vi "get 750 mag stable.vi"(10 "类型":enum16{"temp", "field", "position"}(ring), 11 "输出簇":T1={"initialize"=enum."SR830", "6221"={"6221 Resource"="GPIB0::24::INSTR", "Delta status"=FALSE, "电流|RMS(A)"=0.0}, "SR830+6221"={"source"=0, "Current(A)"=0.0, "阻抗(Ohm)"=0.0, "SR830 1"=FALSE, "SR830 2"=FALSE, "SR830 3"=FALSE, "SR830 4"=FALSE, "VISA 1"="", "VISA 2"="", "VISA 3"="", "VISA 4"="", "Reserve 1"=0, "Reserve 2"=-1, "Reserve 3"=-1, "Reserve 4"=-1, "Sensitivity 1"=-1, "Sensitivity 2"=0, "Sensitivity 3"=-1, "Sensitivity 4"=-1, "量程入 1"=0, "量程入 2"=0, "量程入 3"=0, "量程入 4"=0}, "2400"={"2400"=FALSE, "VISA"="", "Output Level (0)"=1e-05, "Compliance  Level (0.1)"=10.0}, "ch"={"ch"=[], "current"=[], "change?"=[], "holding current\nwhen change ch?"=FALSE}, "Instrument"={"325 Resource "="GPIB0::13::INSTR", "Input (0:A) 325"=0, "Heater Output (1:1) 325"=1, "340 Resource"="GPIB0::14::INSTR", "Input (0:A) 340"=0, "Loop (0: 1)"=0, "Input (0:B) 340"=1, "Loop (1: 1)"=0, "340 Status"=refnum, "Instrument Type"=enum."PPMS-Rotate", "quantum design"=refnum, "semaphore 325"=refnum, "TCP master instance"=refnum, "M24C Resource"="GPIB0::24::INSTR", "4G supply"="GPIB0::24::INSTR", "Temp Status 24C"=refnum, "Temp"=refnum, "9T信号"=refnum, "limit"={"Field limit"=0.0, "Field rate limit"=0.0, "Temp limit"=0.0, "Temp low limit"=0.0, "Temp rate limit "=0.0}, "4g supply status"=refnum, "vi路径"="", "in-plane"="", "out-plane"="", "in-plane signal"=FALSE, "out-plane signal"=FALSE, "in plane 信号"=refnum, "pzt volt"=refnum, "Aborting"=refnum, "数据文件"=refnum, "warning"=refnum, "750 visa"="", "750 rotate"="", "335 Status 2"=refnum, "335 Resource "="GPIB0::24::INSTR", "Input (0:A) 335"=0, "Input (0:B) 335"=1, "Heater Output (1:1) 335"=1, "semaphore 340"=refnum, "semaphore 335"=refnum, "325 Status"=refnum, "semaphore 750"=refnum, "750 field status"=refnum, "camg 振荡状态"=refnum, "列表框"=refnum, "编辑列表框？"=refnum, "camg Rate"=refnum, "行数"=refnum, "TM620"="TCPIP0::192.168.1.5::4266::SOCKET"}, "2614B"={"2614B chA"=FALSE, "2614B chB"=FALSE, "VISA"=""}, "33522b"={"33522b resource name"="", "零电压"=0.0, "最大电压"=148.0, "间隔"=4.0, "最小电压"=-48.0, "PZT Scan?"=FALSE}, "gating type"=enum."2614(daul)", "层数"=0, "行数"=0, "是否处理"=[]} {"Instrument"."Loop (1: 1)" items=["1"=1, "2"=2]; "Instrument"."Loop (0: 1)" items=["1"=1, "2"=2]; "Instrument"."Input (0:B) 340" items=["A", "B", "C", "D"]; "Instrument"."Heater Output (1:1) 335" items=["1"=1, "2"=2]; "Instrument"."Input (0:B) 335" items=["A", "B"]; "Instrument"."Input (0:A) 335" items=["A", "B"]; "Instrument"."Heater Output (1:1) 325" items=["1"=1, "2"=2]; "Instrument"."Input (0:A) 325" items=["A", "B"]; "Instrument"."Input (0:A) 340" items=["1"=1, "2"=2]; "SR830+6221"."Sensitivity 4" items=["Auto Gain"=-1, "2 nV/fA"=0, "5 nV/fA"=1, "10 nV/fA"=2, "20 nV/fA"=3, "50 nV/fA"=4, "100 nV/fA"=5, "200 nV/fA"=6, "500 nV/fA"=7, "1 uV/pA"=8, "2 uV/pA"=9, "5 uV/pA"=10, "10 uV/pA"=11, "20 uV/pA"=12, "50 uV/pA"=13, "100 uV/pA"=14, "200 uV/pA"=15, "500 uV/pA"=16, "1 mV/nA"=17, "2 mV/nA"=18, "5 mV/nA"=19, "10 mV/nA"=20, "20 mV/nA"=21, "50 mV/nA"=22, "100 mV/nA"=23, "200 mV/nA"=24, "500 mV/mA"=25, "1 V/uA"=26]; "SR830+6221"."Sensitivity 3" items=["Auto Gain"=-1, "2 nV/fA"=0, "5 nV/fA"=1, "10 nV/fA"=2, "20 nV/fA"=3, "50 nV/fA"=4, "100 nV/fA"=5, "200 nV/fA"=6, "500 nV/fA"=7, "1 uV/pA"=8, "2 uV/pA"=9, "5 uV/pA"=10, "10 uV/pA"=11, "20 uV/pA"=12, "50 uV/pA"=13, "100 uV/pA"=14, "200 uV/pA"=15, "500 uV/pA"=16, "1 mV/nA"=17, "2 mV/nA"=18, "5 mV/nA"=19, "10 mV/nA"=20, "20 mV/nA"=21, "50 mV/nA"=22, "100 mV/nA"=23, "200 mV/nA"=24, "500 mV/mA"=25, "1 V/uA"=26]; "SR830+6221"."Sensitivity 1" items=["Auto Gain"=-1, "2 nV/fA"=0, "5 nV/fA"=1, "10 nV/fA"=2, "20 nV/fA"=3, "50 nV/fA"=4, "100 nV/fA"=5, "200 nV/fA"=6, "500 nV/fA"=7, "1 uV/pA"=8, "2 uV/pA"=9, "5 uV/pA"=10, "10 uV/pA"=11, "20 uV/pA"=12, "50 uV/pA"=13, "100 uV/pA"=14, "200 uV/pA"=15, "500 uV/pA"=16, "1 mV/nA"=17, "2 mV/nA"=18, "5 mV/nA"=19, "10 mV/nA"=20, "20 mV/nA"=21, "50 mV/nA"=22, "100 mV/nA"=23, "200 mV/nA"=24, "500 mV/mA"=25, "1 V/uA"=26]; "SR830+6221"."Sensitivity 2" items=["Auto Gain"=-1, "2 nV/fA"=0, "5 nV/fA"=1, "10 nV/fA"=2, "20 nV/fA"=3, "50 nV/fA"=4, "100 nV/fA"=5, "200 nV/fA"=6, "500 nV/fA"=7, "1 uV/pA"=8, "2 uV/pA"=9, "5 uV/pA"=10, "10 uV/pA"=11, "20 uV/pA"=12, "50 uV/pA"=13, "100 uV/pA"=14, "200 uV/pA"=15, "500 uV/pA"=16, "1 mV/nA"=17, "2 mV/nA"=18, "5 mV/nA"=19, "10 mV/nA"=20, "20 mV/nA"=21, "50 mV/nA"=22, "100 mV/nA"=23, "200 mV/nA"=24, "500 mV/mA"=25, "1 V/uA"=26]; "SR830+6221"."Reserve 4" items=["Auto Gain"=-1, "2 nV/fA"=0, "5 nV/fA"=1, "10 nV/fA"=2, "20 nV/fA"=3, "50 nV/fA"=4, "100 nV/fA"=5, "200 nV/fA"=6, "500 nV/fA"=7, "1 uV/pA"=8, "2 uV/pA"=9, "5 uV/pA"=10, "10 uV/pA"=11, "20 uV/pA"=12, "50 uV/pA"=13, "100 uV/pA"=14, "200 uV/pA"=15, "500 uV/pA"=16, "1 mV/nA"=17, "2 mV/nA"=18, "5 mV/nA"=19, "10 mV/nA"=20, "20 mV/nA"=21, "50 mV/nA"=22, "100 mV/nA"=23, "200 mV/nA"=24, "500 mV/mA"=25, "1 V/uA"=26]; "SR830+6221"."Reserve 3" items=["Auto Reserve"=-1, "High Reserve"=0, "Normal"=1, "Low Noise"=2]; "SR830+6221"."Reserve 2" items=["Auto Reserve"=-1, "High Reserve"=0, "Normal"=1, "Low Noise"=2]; "SR830+6221"."Reserve 1" items=["Auto Reserve"=-1, "High Reserve"=0, "Normal"=1, "Low Noise"=2]; "SR830+6221"."source" items=["SR830 1", "SR830 2", "SR830 3", "SR830 4"]}) -> (1 "Stable?":bool)   [LabVIEW 2019, in "User lib.lvlib"]
uses:
  User lib.lvlib
  ctl/config.ctl
  <vilib>/NI/Modbus Library/API/Master/Modbus Master.lvclass
  ctl/initialize.ctl
  ctl/Instrument.ctl
  ctl/335 state.ctl
  ctl/Instrument Type.ctl
  lib/QDInstrument.dll
  ctl/limit.ctl
  ctl/9T mag field stauts.ctl
  ctl/warning.ctl
  ctl/Gating type.ctl
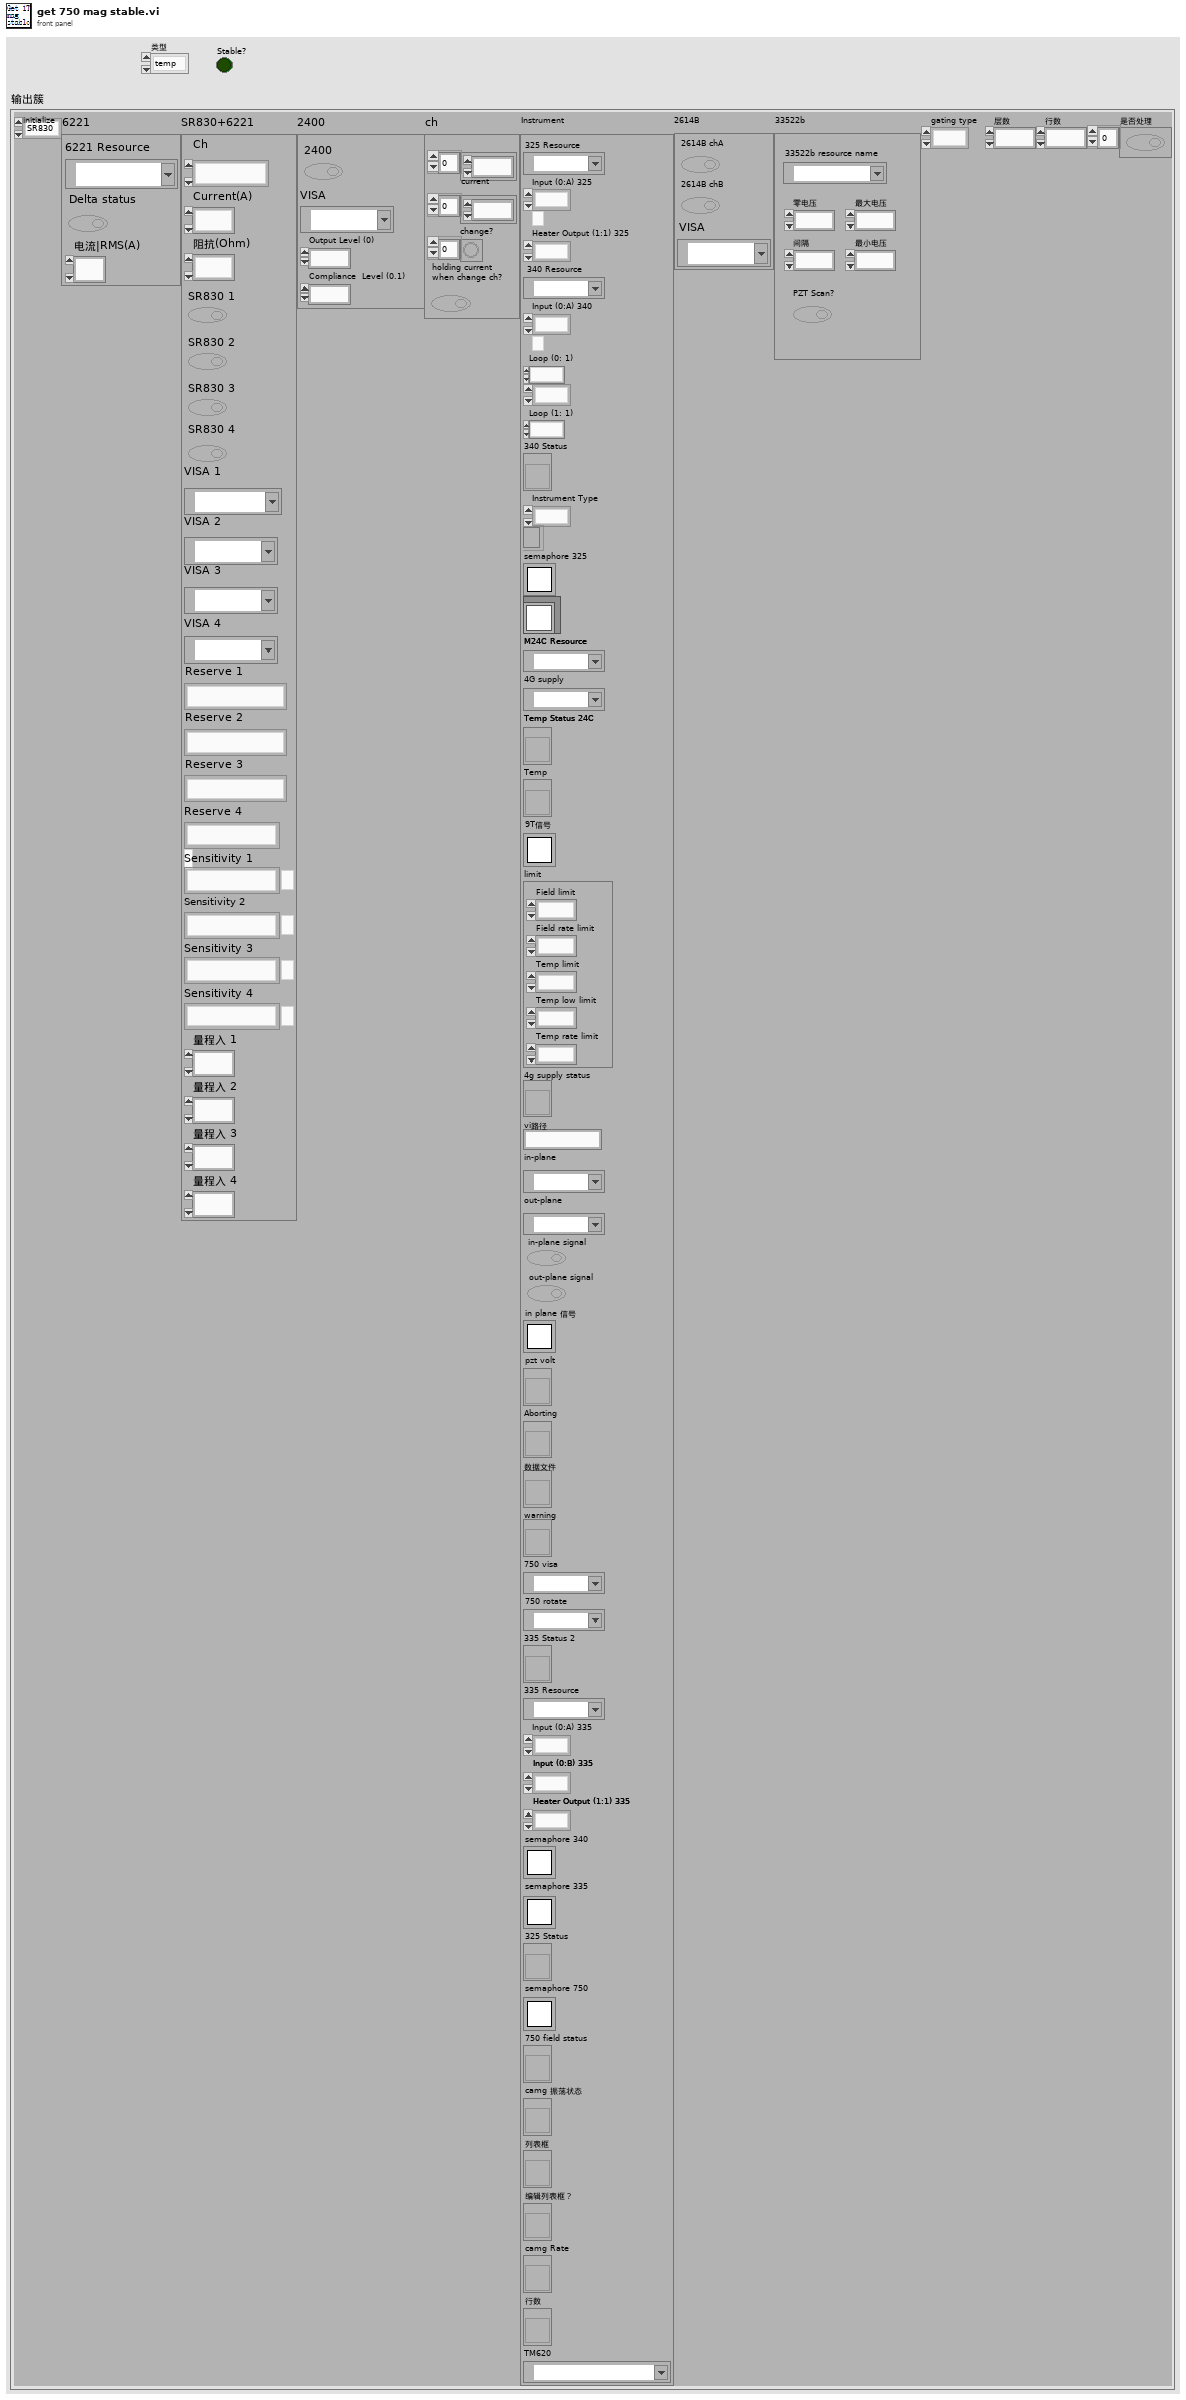
[diagram p1: front panel]
types:
  T1 = typedef "config.ctl" = cluster{"initialize":T2, "6221":cluster{"6221 Resource":refnum<visa-resource-name>, "Delta status":bool, "电流|RMS(A)":dbl}, "SR830+6221":cluster{"source":u16, "Current(A)":dbl, "阻抗(Ohm)":dbl, "SR830 1":bool, "SR830 2":bool, "SR830 3":bool, "SR830 4":bool, "VISA 1":refnum<visa-resource-name>, "VISA 2":refnum<visa-resource-name>, "VISA 3":refnum<visa-resource-name>, "VISA 4":refnum<visa-resource-name>, "Reserve 1":i16, "Reserve 2":i16, "Reserve 3":i16, "Reserve 4":i16, "Sensitivity 1":i16, "Sensitivity 2":i16, "Sensitivity 3":i16, "Sensitivity 4":i16, "量程入 1":i32, "量程入 2":i32, "量程入 3":i32, "量程入 4":i32}, "2400":cluster{"2400":bool, "VISA":refnum<visa-resource-name>, "Output Level (0)":dbl, "Compliance  Level (0.1)":dbl}, "ch":cluster{"ch":i32[], "current":dbl[], "change?":bool[], "holding current\nwhen change ch?":bool}, "Instrument":T3, "2614B":cluster{"2614B chA":bool, "2614B chB":bool, "VISA":refnum<visa-resource-name>}, "33522b":cluster{"33522b resource name":refnum<visa-resource-name>, "零电压":dbl, "最大电压":dbl, "间隔":dbl, "最小电压":dbl, "PZT Scan?":bool}, "gating type":T7, "层数":i32, "行数":i32, "是否处理":bool[]}
  T2 = typedef "initialize.ctl" = enum16{"SR830", "keithley6221-SR830", "Delta", "Delta-tunnelling", "keithley6221-2182-DC", "PZT", "4200"}
  T3 = typedef "Instrument.ctl" = cluster{"325 Resource ":refnum<visa-resource-name>, "Input (0:A) 325":u16, "Heater Output (1:1) 325":u16, "340 Resource":refnum<visa-resource-name>, "Input (0:A) 340":u16, "Loop (0: 1)":u16, "Input (0:B) 340":u16, "Loop (1: 1)":u16, "340 Status":refnum<vi>, "Instrument Type":T4, "quantum design":refnum<k24>, "semaphore 325":T5, "TCP master instance":refnum<class "Modbus Master.lvclass">, "M24C Resource":refnum<visa-resource-name>, "4G supply":refnum<visa-resource-name>, "Temp Status 24C":refnum<vi>, "Temp":refnum<vi>, "9T信号":T5, "limit":T6, "4g supply status":refnum<vi>, "vi路径":string, "in-plane":refnum<visa-resource-name>, "out-plane":refnum<visa-resource-name>, "in-plane signal":bool, "out-plane signal":bool, "in plane 信号":T5, "pzt volt":refnum<vi>, "Aborting":refnum<vi>, "数据文件":refnum<vi>, "warning":refnum<vi>, "750 visa":refnum<visa-resource-name>, "750 rotate":refnum<visa-resource-name>, "335 Status 2":refnum<vi>, "335 Resource ":refnum<visa-resource-name>, "Input (0:A) 335":u16, "Input (0:B) 335":u16, "Heater Output (1:1) 335":u16, "semaphore 340":T5, "semaphore 335":T5, "325 Status":refnum<vi>, "semaphore 750":T5, "750 field status":refnum<vi>, "camg 振荡状态":refnum<vi>, "列表框":refnum<vi>, "编辑列表框？":refnum<vi>, "camg Rate":refnum<vi>, "行数":refnum<vi>, "TM620":refnum<visa-resource-name>}
  T4 = typedef "Instrument Type.ctl" = enum16{"PPMS", "VersaLab", "DynaCool", "SVSM", "PPMS-Rotate", "Lakeshore335", "lengtou2", "9T mag old", "9T cmag", "9T cmag DAC", "9T cmag rotate", "test"}
  T5 = typedef "Semaphore RefNum" = refnum<k1>
  T6 = typedef "limit.ctl" = cluster{"Field limit":dbl, "Field rate limit":dbl, "Temp limit":dbl, "Temp low limit":dbl, "Temp rate limit ":dbl}
  T7 = typedef "Gating type.ctl" = enum32{"null", "2614(daul)", "2400", "6517B"}
  T8 = typedef "335 state.ctl" = u16
  T9 = typedef "9T mag field stauts.ctl" = enum16{"unknow", "Stable", "Sweep up", "Sweep down", "Sweep to zero", "Pause"}
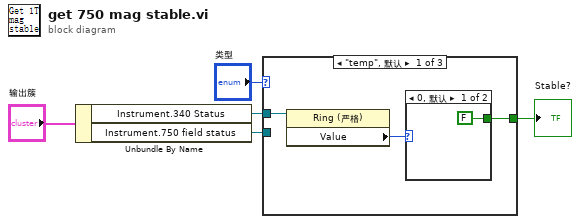
[diagram p0: block diagram]
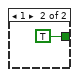
[diagram p2: hidden frame]
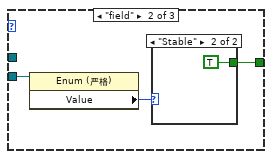
[diagram p3: hidden frame]
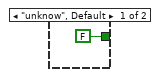
[diagram p4: hidden frame]
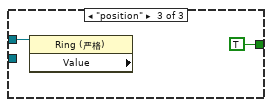
[diagram p5: hidden frame]
diagram:
  n1 = Unbundle By Name("输出簇") -> ("Instrument.340 Status"=w4:refnum<vi>, "Instrument.750 field status"=w3:refnum<vi>)
  n2 = case shown="\"temp\", 默认" "类型" {
    tunnel: w4 -> [w7 _ w17]
    tunnel: w3 -> [_ w13 _]
    tunnel: [w6 w11 TRUE] -> w2
    frame "temp", Default {
      n3 = property class="Ring (严格)"(reference=w7) -> ("Value"=w8:T8)  [unwired: 1 in, 2 out]
      n4 = case shown="0, 默认" w8 {
        tunnel: [FALSE TRUE] -> w6
        frame 0, Default {
        }
        frame 1 {
        }
      }
    }
    frame "field" {
      n5 = property class="Enum (严格)"(reference=w13) -> ("Value"=w12:T9)  [unwired: 1 in, 2 out]
      n6 = case shown="\"Stable\"" w12 {
        tunnel: [FALSE TRUE] -> w11
        frame "unknow", Default {
        }
        frame "Stable" {
        }
      }
    }
    frame "position" {
      n7 = property class="Ring (严格)" props=["Value"](reference=w17) -> ()  [unwired: 1 in, 3 out]
    }
  }
  "Stable?" <- w2
